vi "iCalendar Toolkit Example.vi"(0 "Path to Save":path, 1 "iCalendar File Configuration":T5={"File Name"="Test", "Orginizer Name"="John", "Organizer email"="", "Subject"="John loves LabVIEW", "Location"="Testlocation", "Start Date and Time "=timestamp(3579138000 s since 1904-01-01), "End Date and Time"=timestamp(3579238800 s since 1904-01-01)}, 2 "Sender's Configuration":T3={"Outgoing Mail Server (SMTP)"="smtp.gmail.com", "Port"=587, "Sender's Email"="", "Email Password"="", "Sender's Name"=""}, 5 "error In":errorcluster, 6 "Email Configuration":T1={"Subject"="Checking the Toolkit", "Body"="Please reply!", "Recipients Email Addresses"="", "CC - Optional"=[""]}) -> (14 "ICS Extracted Data":T4, 15 "iCalendar String Out":string, 19 "error out":errorcluster)   [LabVIEW 2016]
doc: "This VI creates a calendar event and sends it via email to the mentioned recipients. After the email is sent the file is being extracted. Also there is an output of the ics format string."
uses:
  controls/ics File Configuration.ctl
  controls/Extract iCalendar String.ctl
  controls/Sender's Configuration.ctl
  controls/Email Configuration.ctl
  controls/Receipants Email Address.ctl
panel:
  in  "Enable?":bool=TRUE
  in  "Enable?":bool=TRUE
  out "Path Out":path caption="Path out"
  # "Instructions:\n1. Fill in the information in Invitation configuration and Email configuration tables.\n2. Make sure that Path to Save, Sender's Gmail ID, Gmail Account Password and Recipients Email Address inputs are entered correctly"
  # "Email Configuration"
  # "Extract Configuration"
  # "Invitation Configuration"
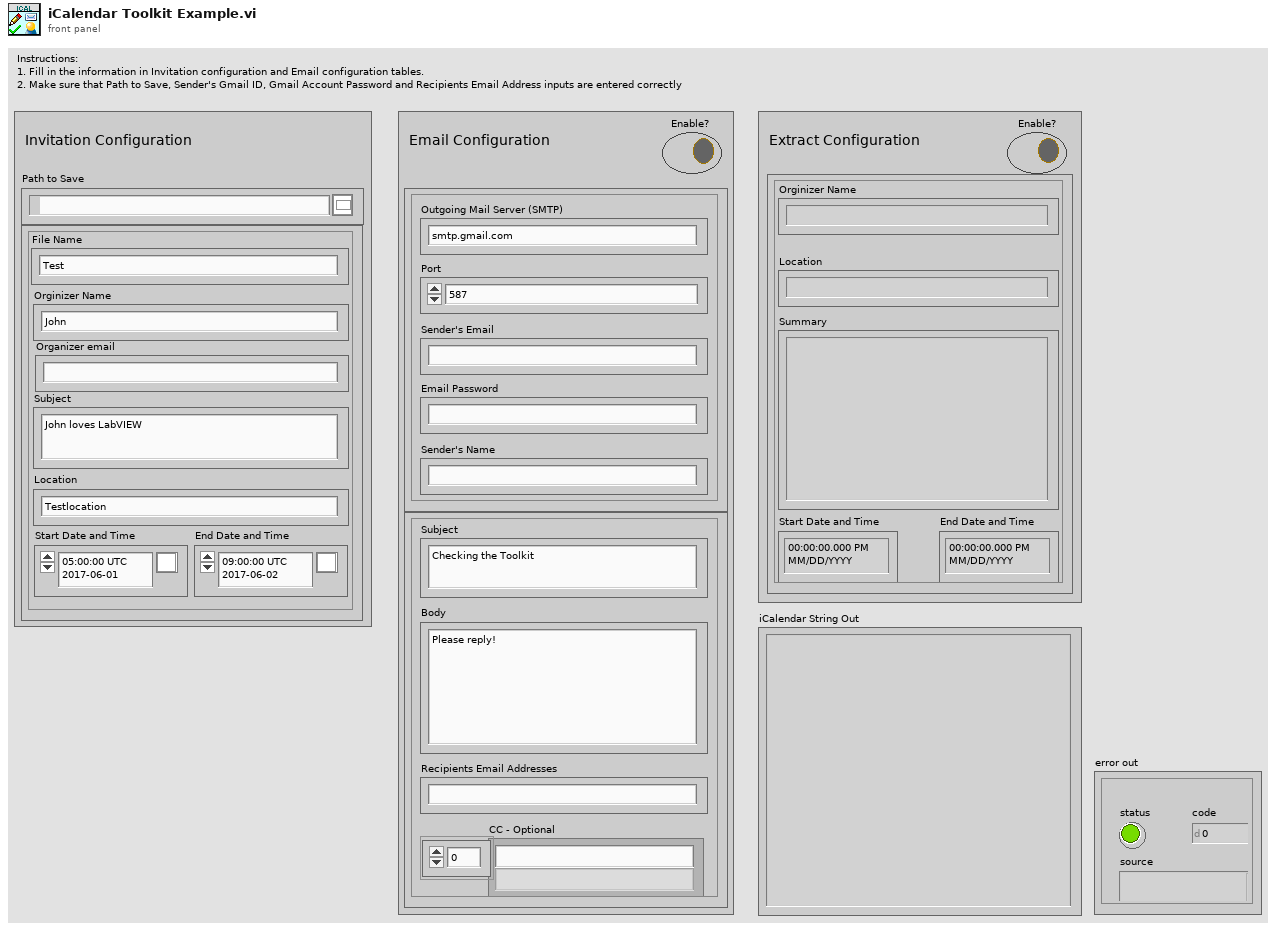
[diagram p1: front panel]
types:
  T1 = typedef "Email Configuration.ctl" = cluster{"Subject":string, "Body":string, "Recipients Email Addresses":T2, "CC - Optional":string[]}
  T2 = typedef "Receipants Email Address.ctl" = string
  T3 = typedef "Sender's Configuration.ctl" = cluster{"Outgoing Mail Server (SMTP)":string, "Port":i32, "Sender's Email":string, "Email Password":string, "Sender's Name":string}
  T4 = typedef "Extract iCalendar string.ctl" = cluster{"Orginizer Name":string, "Location":string, "Summary":string, "Start Date and Time":timestamp, "End Date and Time":timestamp}
  T5 = typedef "ics File Configuration.ctl" = cluster{"File Name":string, "Orginizer Name":string, "Organizer email":string, "Subject":string, "Location":string, "Start Date and Time ":timestamp, "End Date and Time":timestamp}
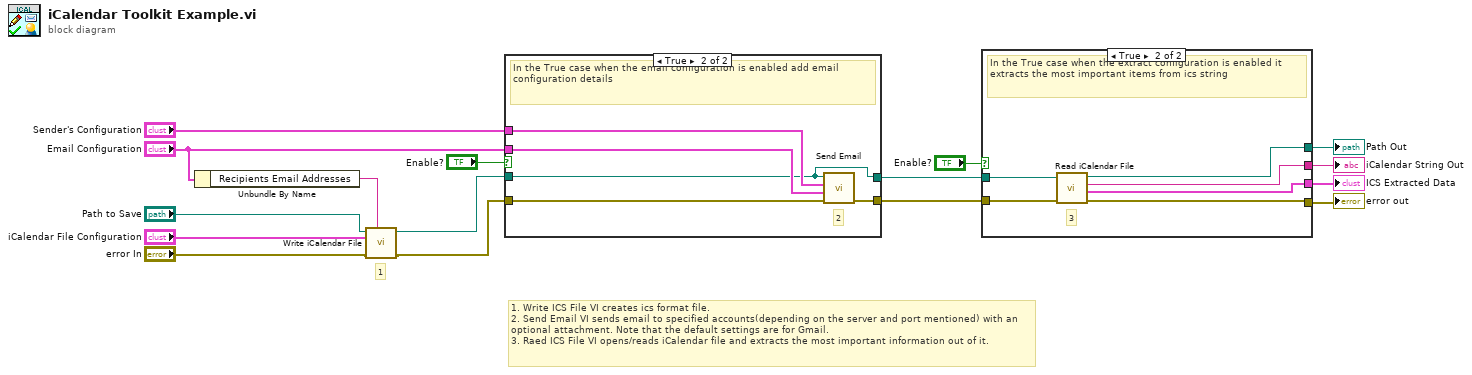
[diagram p0: block diagram]
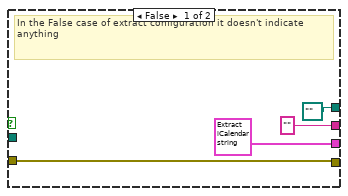
[diagram p2: hidden frame]
diagram:
  # "1"
  # "1. Write ICS File VI creates ics format file. \n2. Send Email VI sends email to specified accounts(depending on the server and port mentioned) with an optional attachment. Note that the default settings are for Gmail. \n3. Raed ICS File VI opens/reads iCalendar file and extracts the most important information out of it."
  n1 = Unbundle By Name("Email Configuration") -> ("Recipients Email Addresses"=w5:T2)
  n2 = call "Write iCalendar File.vi"("Recipient's Email Address"=w5, "error in"="error In", "iCalendar File Configuration"="iCalendar File Configuration", "Path to Save"="Path to Save") -> ("error out"=w9:errorcluster, "Path Out"=w8:path)  [unwired: 6 in]
  n3 = case shown="True" "Enable?" {
    tunnel: w9 -> [w18 w22]
    tunnel: [w18 w23] -> w14
    tunnel: w8 -> [w17 w19]
    tunnel: [w17 w19] -> w3
    tunnel: "Sender's Configuration" -> [_ w20]
    tunnel: "Email Configuration" -> [_ w21]
    frame False {
      # "In the False case of email configuration it doesn't send an email and no details are needed"
    }
    frame True {
      # "2"
      # "In the True case when the email configuration is enabled add email configuration details"
      n4 = call "Send Email.vi"("error in"=w22, "Email Configuration"=w21, "Sender's Configuration"=w20, "Attachment(optional)"=w19) -> ("error out"=w23:errorcluster)  [unwired: 7 in]
    }
  }
  n5 = case shown="True" "Enable?" {
    tunnel: w14 -> [w27 w33]
    tunnel: [w27 w32] -> w13
    tunnel: [T4 {"Orginizer Name"="", "Location"="", "Summary"="", "Start Date and Time"=timestamp(0 s since 1904-01-01), "End Date and Time"=timestamp(0 s since 1904-01-01)} ("Extracted data") w31] -> w4
    tunnel: ["" ("ICS string out") w30] -> w12
    tunnel: [path "" ("Path out") w29] -> w11
    tunnel: w3 -> [_ w28]
    frame False {
      # "In the False case of extract configuration it doesn't indicate anything"
    }
    frame True {
      # "3"
      # "In the True case when the extract configuration is enabled it extracts the most important items from ics string"
      n6 = call "Read iCalendar File.vi"("error in"=w33, "Path to Open"=w28) -> ("error out"=w32:errorcluster, "Extracted Data"=w31:T4, "ICS String Out"=w30:string, "Path Out"=w29:path)  [unwired: 6 in]
    }
  }
  "error out" <- w13
  "iCalendar String Out" <- w12
  "Path Out" <- w11
  "ICS Extracted Data" <- w4
